vi "CaculateProductionYield.vi"(2 "生产统计":T1 {"良率" format="%#.2g"}, 3 "Result(in)":bool) -> (0 "良率统计out":T1 {"良率" format="%#.2g"})   [LabVIEW 2014]
uses:
  Controls/ProductNum.ctl
panel:
  out "1生产统计":T1 {"良率" format="%#.2g"}
  # "%"
  # "%"
  # "%"
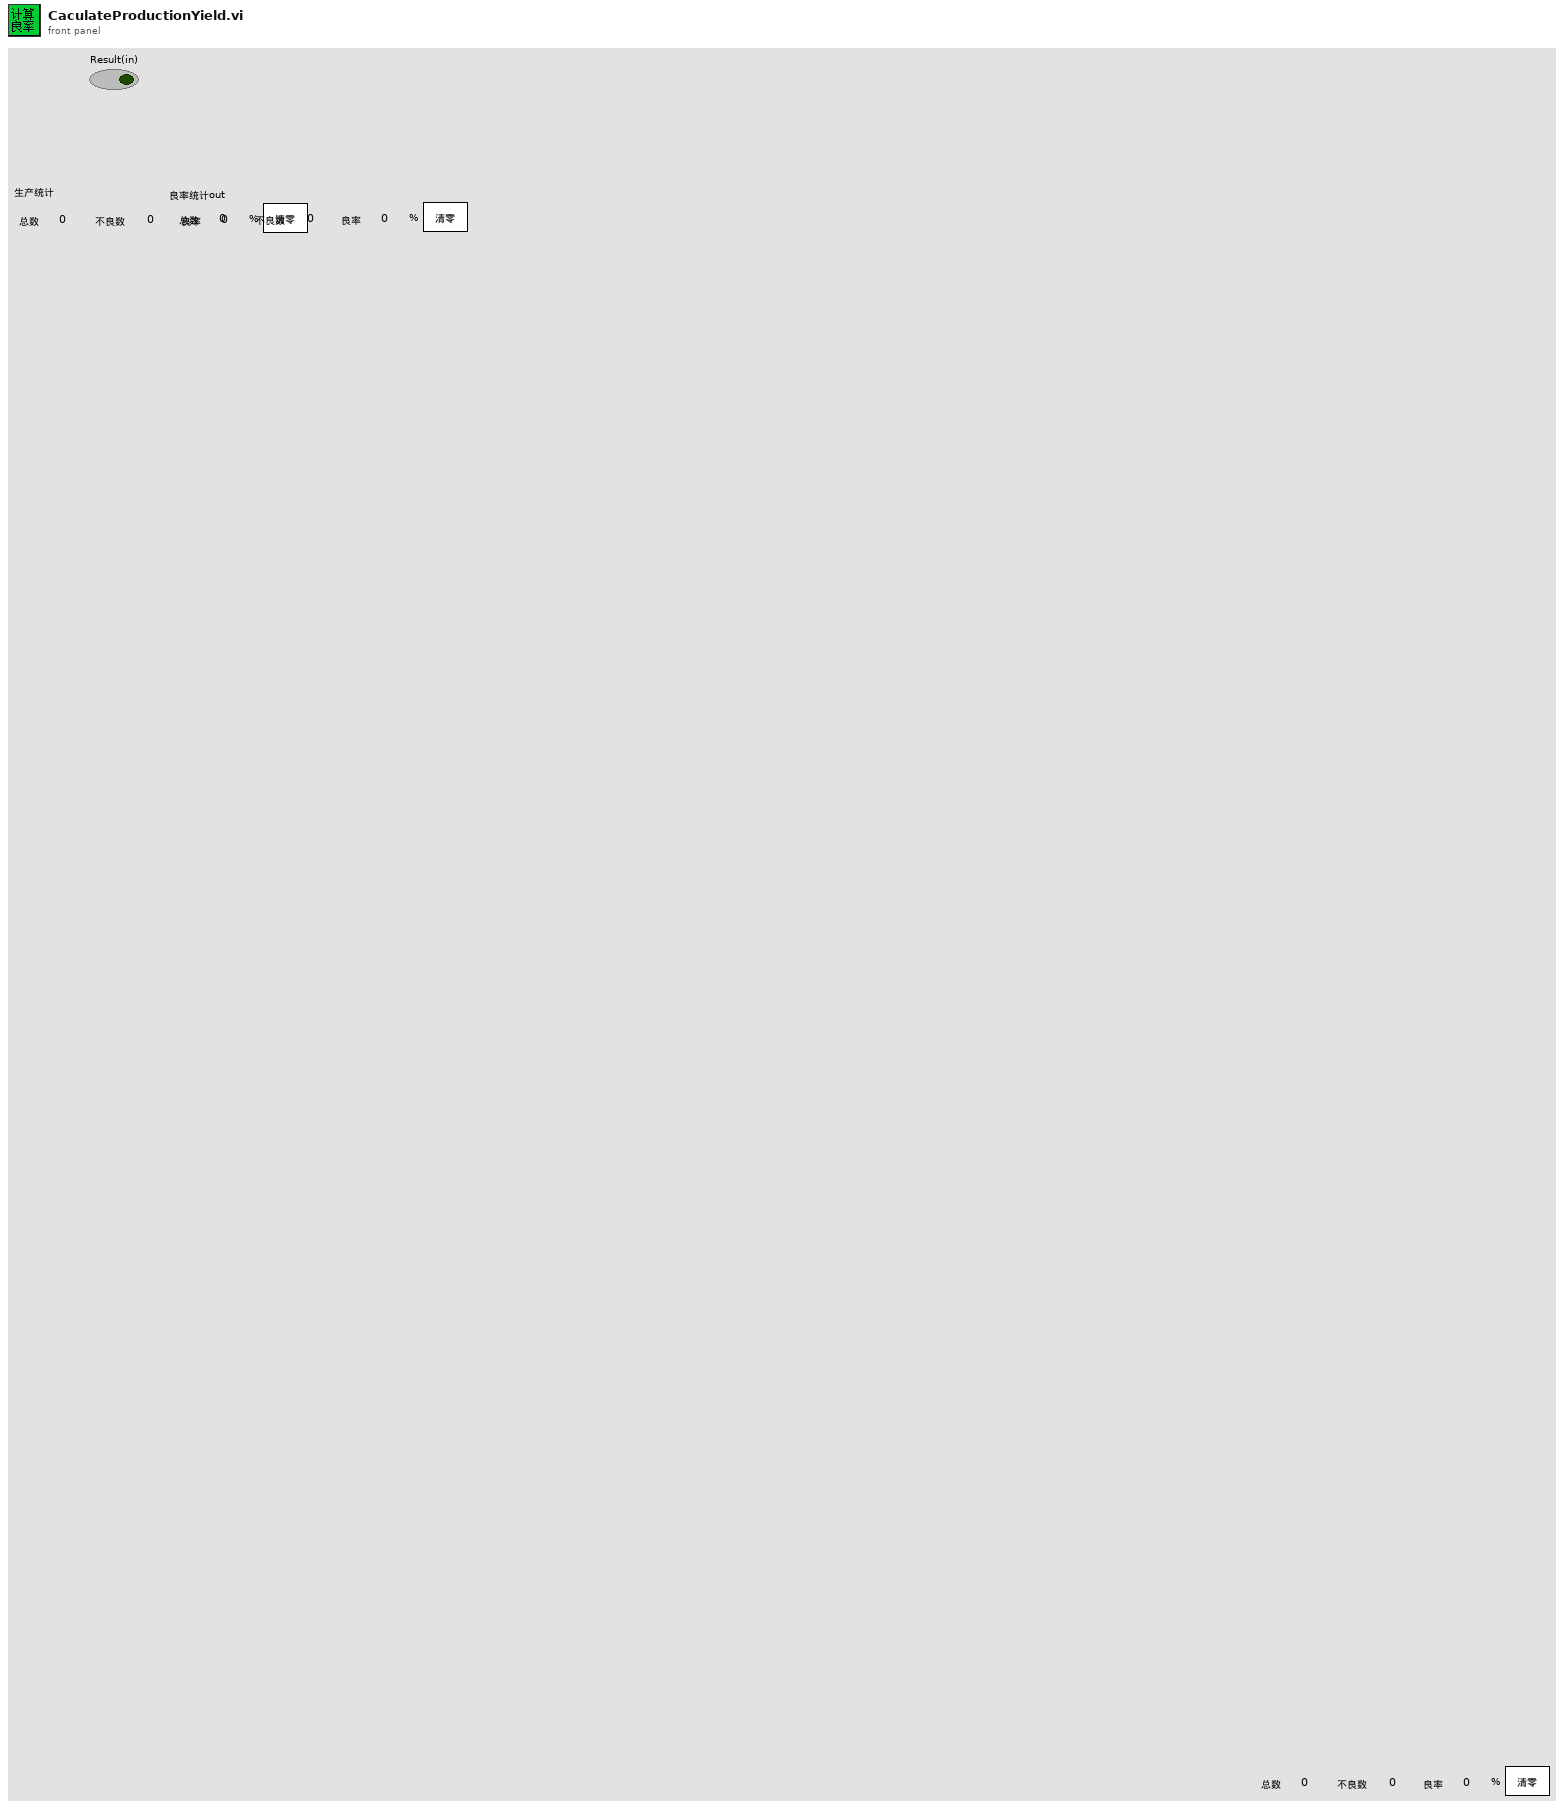
[diagram p1: front panel]
types:
  T1 = typedef "ProductNum.ctl" = cluster{"总数":u64, "不良数":u64, "良率":dbl, "清零":bool}
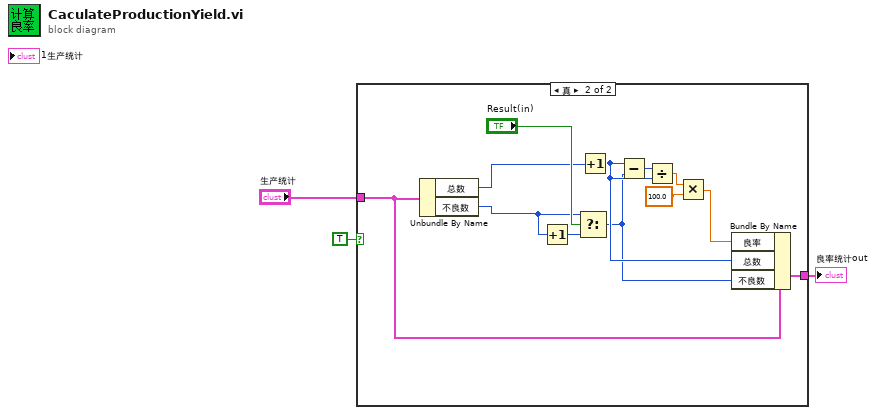
[diagram p0: block diagram]
diagram:
  n1 = case shown="真" TRUE {
    tunnel: "生产统计" -> [w4 w9]
    tunnel: [w4 w8] -> w2
    frame False {
    }
    frame True {
      n2 = Unbundle By Name(w9) -> ("总数"=w11:u64, "不良数"=w10:u64)
      n3 = Increment(x=w10) -> (x+1=w16:u64)
      n4 = Select(t=w10, s="Result(in)", f=w16) -> (s? t:f=w6:u64)
      n5 = Increment(x=w11) -> (x+1=w7:u64)
      n6 = Subtract(x=w7, y=w6) -> (x-y=w12:u64)
      n7 = Divide(x=w12, y=w7) -> (x/y=w13:dbl)
      n8 = Multiply(x=w13, y=100.0) -> (x*y=w5:dbl)
      n9 = Bundle By Name(cluster=w9, "良率"=w5, "总数"=w7, "不良数"=w6) -> (w8:T1)
    }
  }
  "良率统计out" <- w2
